vi "Distance Finder.vi"(0 "Grey in":T2, 5 "Array":T3[](array[typedef]) {"Distance (Real-World)" format="%.2f"; "Location (Real-World)"."Y" format="%.2g"; "Location (Real-World)"."X" format="%.2f"; "Noise" format="%.2f"; "Location (Pixel)"."Y" format="%.2g"; "Location (Pixel)"."X" format="%.2f"; "Strength" format="%.2f"; "Distance (Pixel)" format="%.2f"}, 7 "LL":string[](array[string]), 9 "HL":string[](array[string]), 11 "error in (no error)":errorcluster) -> (4 "RGB out":T2, 10 "Analysis":T1(array[cluster]), 15 "error out":errorcluster)   [LabVIEW 2020]
uses:
  <vilib>/vision/Measure.llb/Edge New.ctl
  <vilib>/vision/Image Controls.llb/IMAQ Image.ctl
panel:
  out "Results 2":string[][](array[string])
  out "Length":dbl[](array[numeric])
  out "logical AND":bool
  out "output array":i32[](array[numeric])
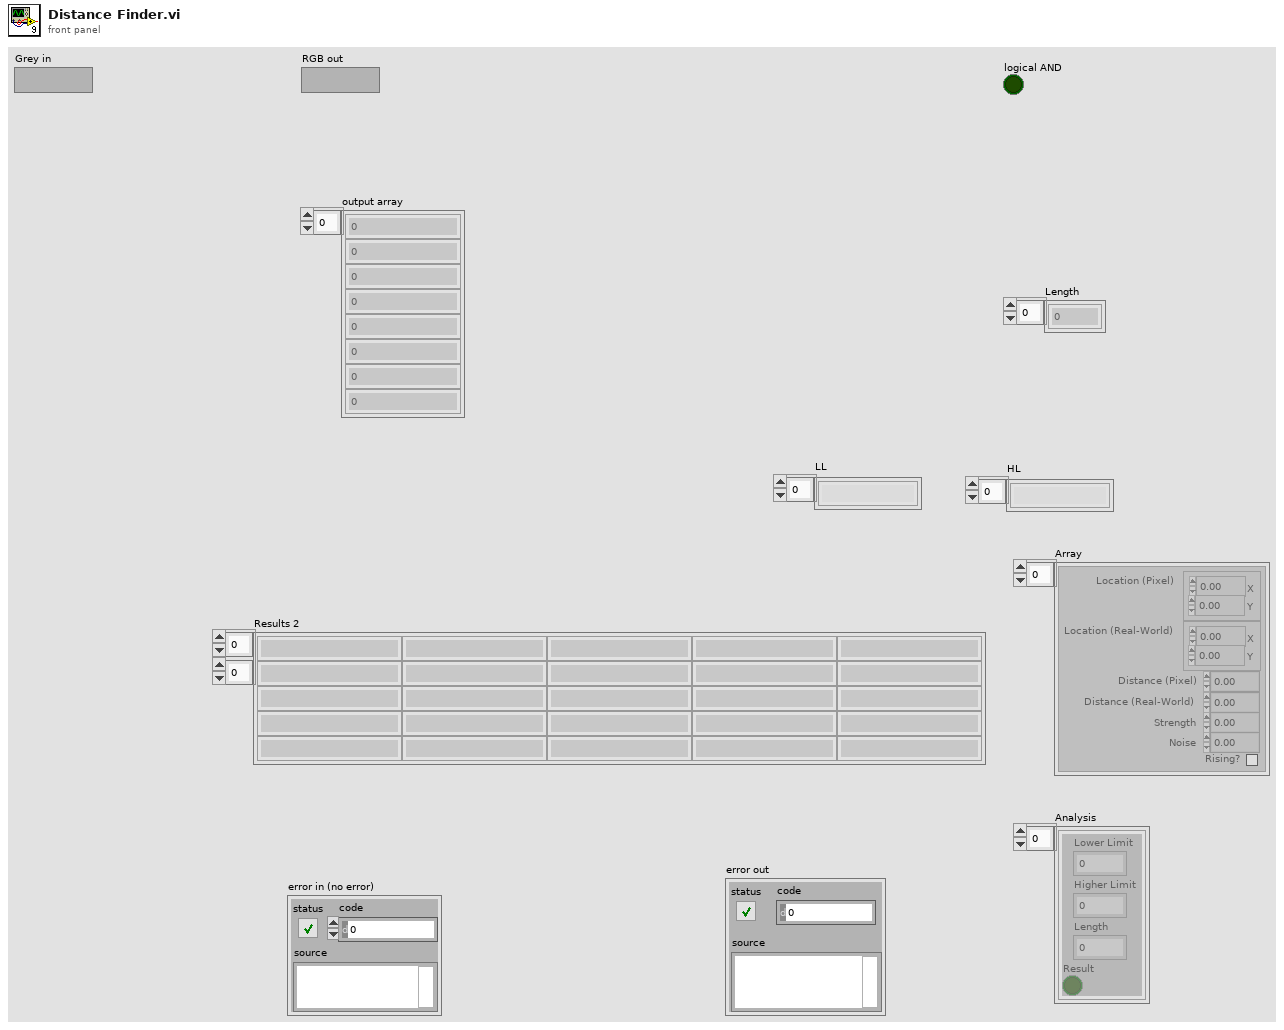
[diagram p1: front panel]
types:
  T1 = cluster{"Lower Limit":dbl, "Higher Limit":dbl, "Length":dbl, "Result":bool}[]
  T2 = typedef "IMAQ Image.ctl" = refnum<image>
  T3 = typedef "Edge New.ctl" = cluster{"Location (Pixel)":cluster{"X":sgl, "Y":sgl}, "Location (Real-World)":cluster{"X":sgl, "Y":sgl}, "Distance (Pixel)":dbl, "Distance (Real-World)":dbl, "Strength":dbl, "Noise":dbl, "Rising?":bool}
  T4 = cluster{i32[], cluster{"Contour Type":u32, "Contour Type":i32, i32[]}[]}
  T5 = cluster{"Contour Type":u32, "Contour Type":i32, i32[]}[]
  T6 = cluster{"Contour Type":u32, "Contour Type":i32, i32[]}
  T7 = cluster{"Lower Limit":dbl, "Higher Limit":dbl, "Length":dbl, "Result":bool}
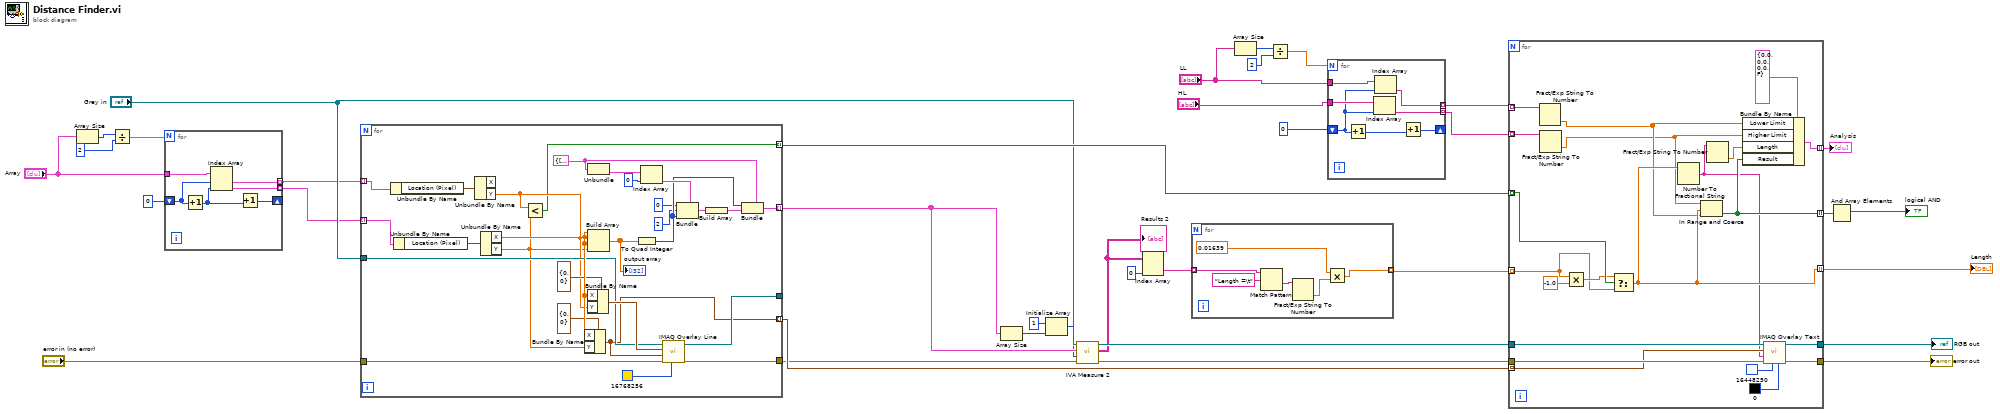
[diagram p0: block diagram]
diagram:
  n1 = Array Size(array="Array") -> (size(s)=w16:i32)
  n2 = Divide(x=w16, y=2) -> (x/y=w15:dbl)
  n3 = for {
    N: w15 -> [_]
    shift-right: [w40] -> _
    shift-left: 0 ("y") -> [w41]
    tunnel: "Array" -> [w39]
    tunnel: [w38] -> w11 mode=indexing
    tunnel: [w37] -> w10 mode=indexing
    n4 = Increment(x=w41) -> (x+1=w42:i32)
    n5 = Index Array(array=w39, index #1=w41, index #2=w42) -> (element #1=w38:T3, element #2=w37:T3)
    n6 = Increment(x=w42) -> (x+1=w40:i32)
  }
  n7 = for {
    tunnel: "Grey in" -> [w47]
    tunnel: [w53] -> _
    tunnel: [w52] -> w25 mode=indexing
    tunnel: w10 -> [w51] mode=indexing
    tunnel: "error in (no error)" -> [w50]
    tunnel: [w49] -> w31
    tunnel: w11 -> [w48] mode=indexing
    tunnel: [w46] -> w33 mode=indexing
    tunnel: [w43] -> w27 mode=indexing
    w63 = T4 {[], [{"Contour Type"=0, "Contour Type"=2, []}]} ("element")
    n8 = Unbundle By Name(w48) -> ("Location (Pixel)"=w70:cluster{"X":sgl, "Y":sgl})
    n9 = Unbundle By Name(w51) -> ("Location (Pixel)"=w69:cluster{"X":sgl, "Y":sgl})
    n10 = Unbundle By Name(w70) -> ("Y"=w45:sgl)  [unwired: 1 out]
    n11 = Unbundle By Name(w69) -> ("X"=w58:sgl, "Y"=w44:sgl)
    n12 = Less?(x=w45, y=w44) -> (x < y?=w43:bool)
    n13 = Bundle By Name(cluster=cluster{"X":i32, "Y":i32} {"X"=0, "Y"=0} ("End Point"), "X"=w58, "Y"=w44) -> (w46:cluster{"X":i32, "Y":i32})
    n14 = Unbundle(w63) -> (w68:T5)  [unwired: 1 out]
    n15 = Build Array(w58, w45, w58, w44) -> (w62:sgl[])
    "output array" <- w62
    n16 = Bundle By Name(cluster=cluster{"X":i32, "Y":i32} {"X"=0, "Y"=0} ("End Point"), "X"=w58, "Y"=w45) -> (w54:cluster{"X":i32, "Y":i32})
    n17 = To Quad Integer(1:w62) -> (0:w61:i64[])
    n18 = Index Array(array=w68, index=0) -> (element=w65:T6)
    n19 = call "IMAQ Overlay Line"("Color"=u32 16768256, "error in (no error)"=w50, "End Point"=w46, "Start Point"=w54, "Image"=w47) -> ("error out"=w49:errorcluster, "Image Out"=w53:T2)  [unwired: 5 in]
    n20 = Bundle(cluster=w65, "Contour Type"=u32 0, "Contour Type"=2, w61) -> (w64:T6)
    n21 = Build Array(w64) -> (w67:T5)
    n22 = Bundle(cluster=w63, w61, w67) -> (w52:T4)
  }
  n23 = Array Size(array=w25) -> (size(s)=w19:i32)
  n24 = Initialize Array(1, w19) -> (w18:i32[])
  n25 = call <vilib>:"IVA Measure 2.vi"("error in (no error)"=w31, "Measurements"=w18, "ROI Descriptors"=w25, "Image In"="Grey in") -> ("error out"=w30:errorcluster, "Results"=w21:string[][], "Image Out"=w24:T2)  [unwired: 1 in, 4 out]
  "Results 2" <- w21
  n26 = Index Array(array=w21, index (col)=0 ("disabled index (col)")) -> (element=w17:string[])  [unwired: 1 in]
  n27 = for {
    tunnel: w17 -> [w74] mode=indexing
    tunnel: [w71] -> w23 mode=indexing
    n28 = Match Pattern(string=w74, regular expression="Length =\t") -> (after substring=w76:string)  [unwired: 1 in, 3 out]
    n29 = Fract/Exp String To Number(string=w76) -> (number=w73:dbl)  [unwired: 3 in, 1 out]
    n30 = Multiply(x=0.01639, y=w73) -> (x*y=w71:dbl)
  }
  n31 = Array Size(array="LL") -> (size(s)=w7:i32)
  n32 = Divide(x=w7, y=2) -> (x/y=w5:dbl)
  n33 = for {
    N: w5 -> [_]
    shift-right: [w83] -> _
    shift-left: 0 ("y") -> [w78]
    tunnel: "HL" -> [w80]
    tunnel: [w81] -> w3 mode=indexing
    tunnel: "LL" -> [w79]
    tunnel: [w77] -> w2 mode=indexing
    n34 = Increment(x=w78) -> (x+1=w82:i32)
    n35 = Index Array(array=w80, index=w78) -> (element=w81:string)
    n36 = Index Array(array=w79, index=w78) -> (element=w77:string)
    n37 = Increment(x=w82) -> (x+1=w83:i32)
  }
  n38 = for {
    tunnel: [w103] -> w9 mode=indexing
    tunnel: [w102] -> w35 mode=indexing
    tunnel: w24 -> [w101]
    tunnel: w30 -> [w100]
    tunnel: [w99] -> w34
    tunnel: w33 -> [w98] mode=indexing
    tunnel: [w95] -> w32
    tunnel: [w93] -> w28 mode=indexing
    tunnel: w27 -> [w94] mode=indexing
    tunnel: w23 -> [w90] mode=indexing
    tunnel: w2 -> [w87] mode=indexing
    tunnel: w3 -> [w86] mode=indexing
    n39 = Fract/Exp String To Number(string=w87) -> (number=w89:dbl)  [unwired: 3 in, 1 out]
    n40 = Fract/Exp String To Number(string=w86) -> (number=w88:dbl)  [unwired: 3 in, 1 out]
    n41 = Multiply(x=w90, y=-1.0) -> (x*y=w91:dbl)
    n42 = Select(t=w91, s=w94, f=w90) -> (s? t:f=w93:dbl)
    n43 = Number To Fractional String(number=w93) -> (F-format string=w85:string)  [unwired: 3 in]
    n44 = In Range and Coerce(upper limit=w88, x=w93, lower limit=w89) -> (In Range?=w102:bool)  [unwired: 1 out]
    n45 = Fract/Exp String To Number(string=w85) -> (number=w84:dbl)  [unwired: 3 in, 1 out]
    n46 = Bundle By Name(cluster=T7 {"Lower Limit"=0.0, "Higher Limit"=0.0, "Length"=0.0, "Result"=FALSE} ("Cluster"), "Lower Limit"=w89, "Higher Limit"=w88, "Length"=w84, "Result"=w102) -> (w103:T7)
    n47 = call "IMAQ Overlay Text"("BG Color (Transparent)"=u32 0, "Text Color (black)"=u32 16448250, "error in (no error)"=w100, "String"=w85, "Origin"=w98, "Image"=w101) -> ("error out"=w99:errorcluster, "Image Out"=w95:T2)  [unwired: 4 in]
  }
  "error out" <- w34
  "RGB out" <- w32
  "Length" <- w28
  "Analysis" <- w9
  n48 = And Array Elements(Boolean array=w35) -> (logical AND=→"logical AND":bool)
